vi "Log HTTP Request.vi"(6 "Error information":string[](array[string]), 8 "error in":errorcluster, 11 "LabVIEW Web Service Request":refnum<class "Web Request.lvclass">) -> (0 "error out":errorcluster, 3 "LabVIEW Web Service Request out":refnum<class "Web Request.lvclass">)   [LabVIEW 2020, in "WSsupport.lvlib"]
uses:
  WSsupport.lvlib
  <vilib>/wsapi/Web Request.lvclass
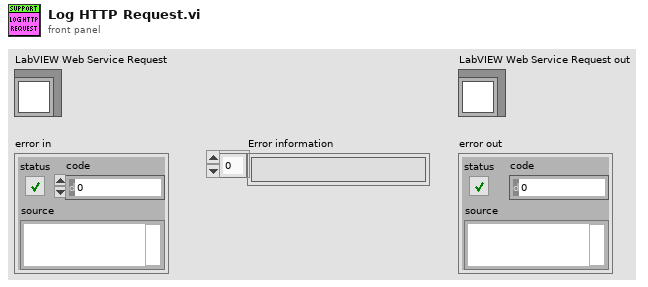
[diagram p1: front panel]
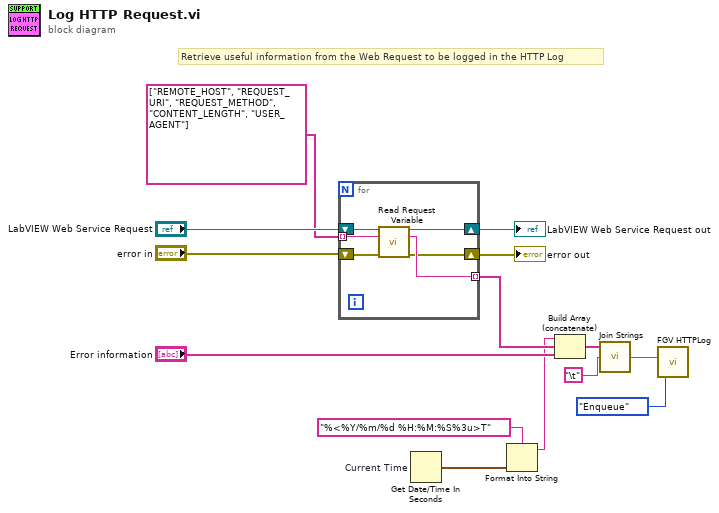
[diagram p0: block diagram]
diagram:
  # "Retrieve useful information from the Web Request to be logged in the HTTP Log"
  n1 = for {
    tunnel: string[] ["REMOTE_HOST", "REQUEST_URI", "REQUEST_METHOD", "CONTENT_LENGTH", "USER_AGENT"] ("variable name") -> [w18] mode=indexing
    shift-right: [w19] -> w13
    shift-left: "LabVIEW Web Service Request" -> [w20]
    tunnel: [w17] -> w9 mode=indexing
    shift-right: [w16] -> w10
    shift-left: "error in" -> [w15]
    n2 = call <vilib>:"Read Request Variable.vi"("LabVIEW Web Service Request"=w20, "variable name"=w18, "error in (no error)"=w15) -> ("LabVIEW Web Service Request out"=w19:refnum<class "Web Request.lvclass">, "value"=w17:string, "error out"=w16:errorcluster)  [unwired: 10 in]
  }
  "LabVIEW Web Service Request out" <- w13
  "error out" <- w10
  n3 = Get Date/Time In Seconds "Current Time"() -> (seconds since 1Jan1904=w6:timestamp)
  n4 = Format Into String(format string="%<%Y/%m/%d %H:%M:%S%3u>T", w6) -> (resulting string=w5:string)  [unwired: 2 in, 1 out]
  n5 = Build Array (concatenate)(w5, w9, "Error information") -> (w4:string[])
  n6 = call <vilib>:"Join Strings.vi"("Separator (,)"="\t", "Strings In"=w4) -> ("String"=w2:string)  [unwired: 1 in]
  n7 = call "FGV HTTPLog.vi"("Action"=enum16{"Reset", "Enqueue", "Dequeue"}."Enqueue", "String to log"=w2) -> ()  [unwired: 1 in, 1 out]
